vi "Read Distance Ultrasonic.vi"(1 "error out":errorcluster, 2 "I2CDevRef":T1 {"Device Address" format="%.0x"}) -> (0 "Inch":dbl)   [LabVIEW 2013]
uses:
  <vilib>/Rock Robotics/WPI/I2C/WPI_I2CDevRef.ctl
  <vilib>/Rock Robotics/SystemInterfaces/Typedef/FPGA_TypedefDigitalModule.ctl
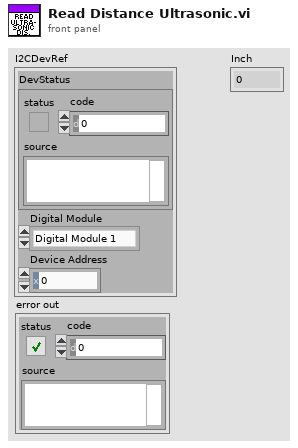
[diagram p1: front panel]
types:
  T1 = typedef "WPI_I2CDevRef.ctl" = cluster{"DevStatus":errorcluster, "Digital Module":T2, "Device Address":u8}
  T2 = typedef "FPGA_TypedefDigitalModule.ctl" = enum16{"Digital Module 1", "Digital Module 2"}
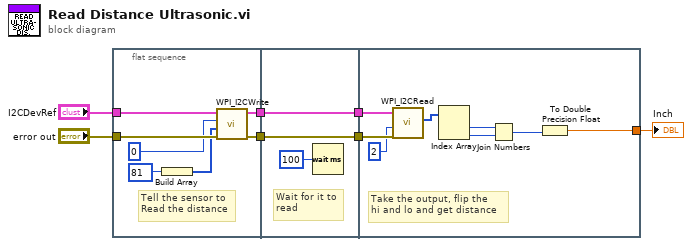
[diagram p0: block diagram]
diagram:
  n1 = flat-sequence {
    tunnel: "I2CDevRef" -> [w14]
    tunnel: "error out" -> [w13]
    tunnel: [w9] -> w7
    tunnel: [w8] -> w6
    tunnel: [w16] -> w5
    tunnel: w7 -> [w16]
    tunnel: [w15] -> w4
    tunnel: w6 -> [w15]
    tunnel: w5 -> [w25]
    tunnel: w4 -> [w24]
    tunnel: [w21] -> w1
    frame #0 {
      # "Tell the sensor to\nRead the distance"
      n2 = Build Array(u8 81) -> (w10:u8[])
      n3 = call <vilib>:"WPI_I2CWrite.vi"("error in (no error)"=w13, "I2CDataToSend"=w10, "I2CRegister"=u8 0, "I2CDevRef"=w14) -> ("error out"=w8:errorcluster, "I2CDevRef"=w9:T1)  [unwired: 6 in]
    }
    frame #1 {
      # "Wait for it to\nread"
      n4 = Wait (ms)(milliseconds to wait=u32 100) -> ()  [unwired: 1 out]
    }
    frame #2 {
      # "Take the output, flip the\nhi and lo and get distance"
      n5 = call <vilib>:"WPI_I2CRead.vi"("error in (no error)"=w24, "I2CBytesToRead"=u8 2, "I2CDevRef"=w25) -> ("Data Out"=w22:u8[])  [unwired: 6 in, 2 out]
      n6 = Index Array(array=w22) -> (element #1=w19:u8, element #2=w18:u8)  [unwired: 2 in]
      n7 = Join Numbers(hi=w19, lo=w18) -> ((hi.lo)=w20:u16)
      n8 = To Double Precision Float(number=w20) -> (double precision float=w21:dbl)
    }
  }
  "Inch" <- w1
